vi "convert_to_base.vi"(7 "unit_set":variant, 8 "error in (no error)":errorcluster, 10 "unit in":string, 11 "value in":dbl) -> (0 "error out":errorcluster, 3 "value out":dbl)   [LabVIEW 2015, in "lv-unit-conversion.lvlib"]
uses:
  lv-unit-conversion.lvlib
  _controls/error.ctl
  _controls/unit_set.ctl
panel:
  out "unit out":string
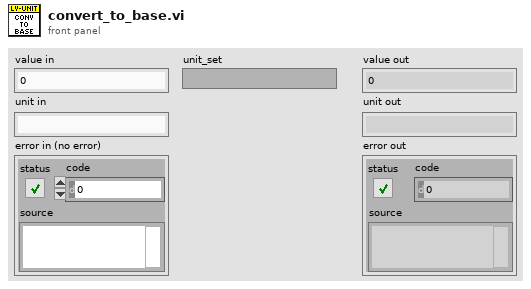
[diagram p1: front panel]
types:
  T1 = typedef "lv-unit-conversion.lvlib/error.ctl" = enum16{"<lv-unit-conversion_error>", "unit_not_found", "xml_parser", "set_not_found", "<null>"}
  T2 = typedef "lv-unit-conversion.lvlib/unit_set.ctl" = cluster{"symbol":string, "name":string, "dimension":string, "is_si_unit":bool, "category":string, "base_unit":string, "conversion_reference":string, "is_exact":bool, "a":dbl, "b":dbl, "c":dbl, "d":dbl, "underlying_def":string, "description":string}
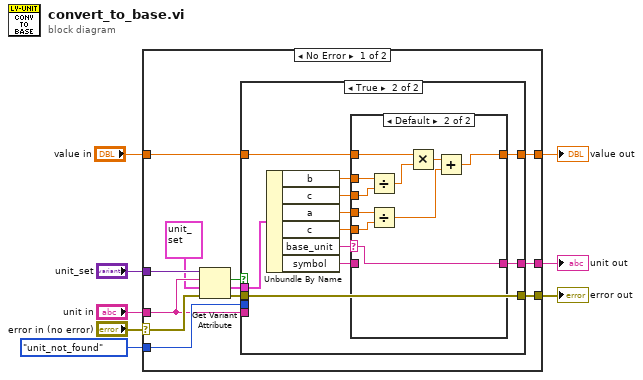
[diagram p0: block diagram]
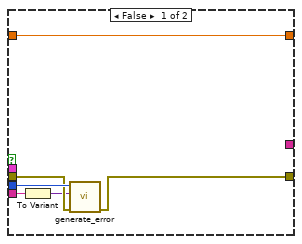
[diagram p2: hidden frame]
diagram:
  n1 = case shown="No Error" "error in (no error)" {
    selector: "error in (no error)" -> [w19 w50]
    tunnel: "unit_set" -> [w20 _]
    tunnel: "value in" -> [w17 _]
    tunnel: [w16 _] -> w5
    tunnel: [w15 _] -> w4
    tunnel: [w12 w50] -> w3
    tunnel: error."unit_not_found" ("error") -> [w11 _]
    tunnel: "unit in" -> [w10 _]
    frame No Error {
      n2 = Get Variant Attribute(Variant=w20, name=w10, default value (empty Variant)=T2 {"symbol"="", "name"="", "dimension"="", "is_si_unit"=FALSE, "category"="", "base_unit"="", "conversion_reference"="", "is_exact"=FALSE, "a"=0.0, "b"=0.0, "c"=0.0, "d"=0.0, "underlying_def"="", "description"=""} ("unit_set"), error in=w19) -> (found=w14:bool, value=w18:T2, error out=w13:errorcluster)  [unwired: 1 out]
      n3 = case shown="True" w14 {
        tunnel: w18 -> [_ w37]
        tunnel: w17 -> [w21 w36]
        tunnel: [w21 w35] -> w16
        tunnel: [_ w28] -> w15
        tunnel: w13 -> [w25 w27]
        tunnel: [w24 w27] -> w12
        tunnel: w11 -> [w26 _]
        tunnel: w10 -> [w23 _]
        frame False {
          n4 = To Variant(anything=w23) -> (Variant=w22:variant)
          n5 = call "generate_error.vi"("error in (no error)"=w25, "data"=w22, "error"=w26) -> ("error out"=w24:errorcluster)  [unwired: 8 in]
        }
        frame True {
          n6 = Unbundle By Name(w37) -> ("b"=w34:dbl, "c"=w33:dbl, "a"=w32:dbl, "c"=w31:dbl, "base_unit"=w30:string, "symbol"=w29:string)
          n7 = case shown="Default" w30 {
            selector: w30 -> [_ w40]
            tunnel: w36 -> [w39 w48]
            tunnel: [w39 w45] -> w35
            tunnel: w34 -> [_ w44]
            tunnel: w33 -> [_ w43]
            tunnel: w32 -> [_ w42]
            tunnel: w31 -> [_ w41]
            tunnel: w29 -> [w38 _]
            tunnel: [w38 w40] -> w28
            frame "" {
            }
            frame Default {
              n8 = Divide(x=w44, y=w43) -> (x/y=w49:dbl)
              n9 = Divide(x=w42, y=w41) -> (x/y=w46:dbl)
              n10 = Multiply(x=w48, y=w49) -> (x*y=w47:dbl)
              n11 = Add(x=w47, y=w46) -> (x+y=w45:dbl)
            }
          }
        }
      }
    }
    frame Error {
    }
  }
  "value out" <- w5
  "error out" <- w3
  "unit out" <- w4
